vi "skipComment.vi"(11 "Content":string[](array[string])) -> (3 "Content":string[](array[string]))   [LabVIEW 2016]
doc: "Skip the comment (#) and empty line in the text array."
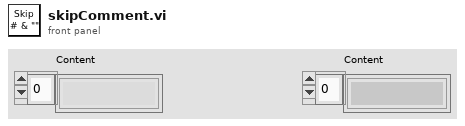
[diagram p1: front panel]
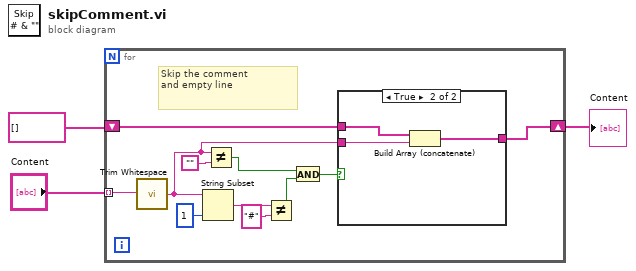
[diagram p0: block diagram]
diagram:
  n1 = for {
    tunnel: "Content" -> [w10] mode=indexing
    shift-right: [w5] -> w2
    shift-left: string[] [] -> [w4]
    # "Skip the comment\nand empty line"
    n2 = call <vilib>:"Trim Whitespace.vi"("string"=w10) -> ("trimmed string"=w6:string)  [unwired: 1 in]
    n3 = String Subset(string=w6, length (rest)=1 ("length (rest)")) -> (substring=w13:string)  [unwired: 1 in]
    n4 = Not Equal?(x=w6, y="") -> (x != y?=w9:bool)
    n5 = Not Equal?(x=w13, y="#") -> (x != y?=w8:bool)
    n6 = And(x=w9, y=w8) -> (x .and. y?=w7:bool)
    n7 = case shown="True" w7 {
      tunnel: w6 -> [_ w18]
      tunnel: [w15 w17] -> w5
      tunnel: w4 -> [w15 w16]
      frame False {
      }
      frame True {
        n8 = Build Array (concatenate)(w16, w18) -> (w17:string[])
      }
    }
  }
  "Content" <- w2
